vi "全局 1.vi"() -> ()   [LabVIEW 2020]
panel:
  out "工位2逆向磨合开始时间":u32
  out "工位1逆向磨合开始时间":u32
  out "工位2正向磨合结束时间":dbl
  out "工位2正向磨合开始时间":u32
  out "工位1正向磨合结束时间":dbl
  out "工位1正向磨合开始时间":u32
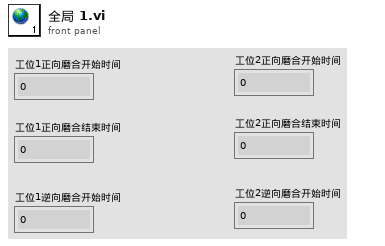
[diagram p1: front panel]
diagram:
